vi "Save lineouts.vi"(10 "Path":path, 11 "Point Grey Camera in":refnum<class "Point Grey Camera.lvclass">) -> ()   [LabVIEW 2020, in "Point Grey Camera.lvclass"]
uses:
  Point Grey Camera.lvclass
  Point Grey Camera.lvclass/Point Grey Camera.ctl
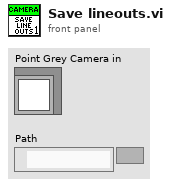
[diagram p1: front panel]
types:
  T1 = typedef "OnOffTypeDef.ctl" = enum16{"off", "on"}
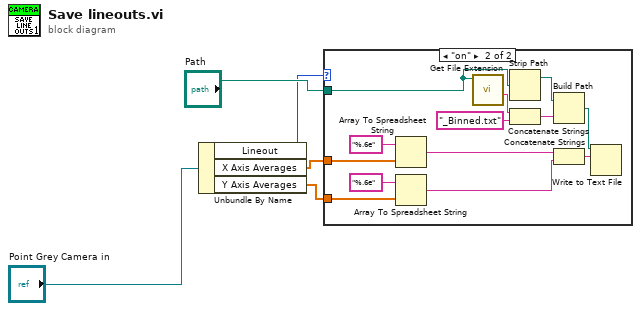
[diagram p0: block diagram]
diagram:
  n1 = Unbundle By Name("Point Grey Camera in") -> ("Lineout"=w1:T1, "X Axis Averages"=w2:sgl[], "Y Axis Averages"=w3:sgl[])
  n2 = case shown="\"on\"" w1 {
    tunnel: "Path" -> [_ w13]
    tunnel: w2 -> [_ w11]
    tunnel: w3 -> [_ w9]
    frame "off", Default {
    }
    frame "on" {
      n3 = Array To Spreadsheet String(array=w11, 3:"%.6e" ("format string")) -> (spreadsheet string=w8:string)  [unwired: 1 in]
      n4 = Array To Spreadsheet String(array=w9, 3:"%.6e" ("format string")) -> (spreadsheet string=w7:string)  [unwired: 1 in]
      n5 = call <vilib>:"Get File Extension.vi"("file"=w13) -> ("filename without extension"=w17:string)  [unwired: 6 in, 4 out]
      n6 = Strip Path(path=w13) -> (stripped path=w15:path)  [unwired: 1 out]
      n7 = Concatenate Strings(w17, "_Binned.txt" ("string")) -> (w16:string)
      n8 = Build Path(base path=w15, name or relative path=w16) -> (appended path=w18:path)
      n9 = Concatenate Strings(w8, w7) -> (w6:string)
      n10 = Write to Text File(file (use dialog)=w18, text=w6) -> ()  [unwired: 2 in, 3 out]
    }
  }
